vi "Check Trigger.vi"(3 "error in (no error)":errorcluster, 4 "Average Integration\nThreshold (V ms)":dbl(slide)=100.0 scale=0.0..100.0, 5 "Force Trigger":bool, 6 "Signals":waveform(dbl)[](array[waveform])) -> (0 "error out":errorcluster, 1 "Average Raw Signal\n Integration Value":dbl, 2 "Triggered":bool)   [LabVIEW 2013]
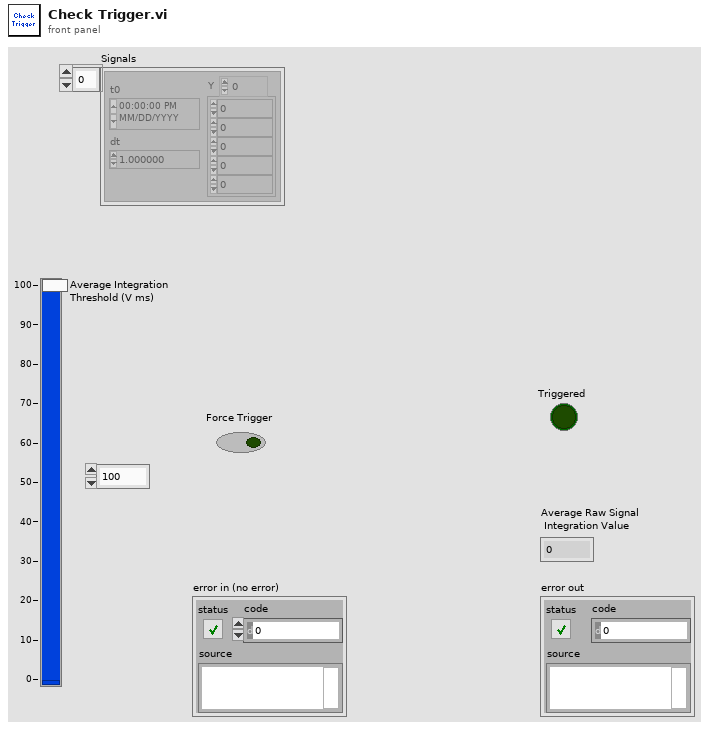
[diagram p1: front panel]
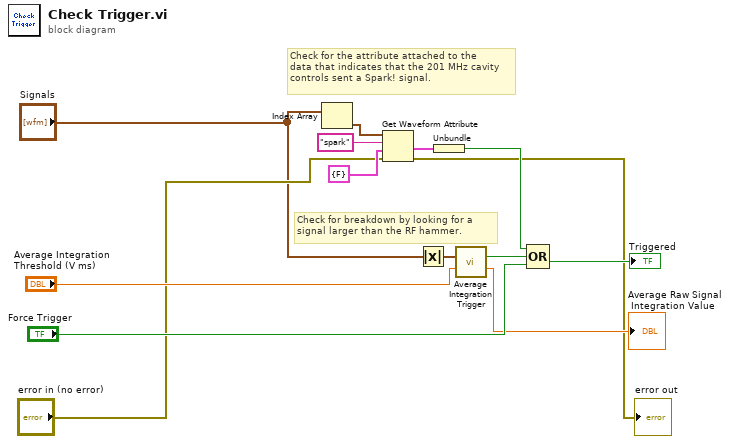
[diagram p0: block diagram]
diagram:
  # "Check for the attribute attached to the\ndata that indicates that the 201 MHz cavity\ncontrols sent a Spark! signal."
  # "Check for breakdown by looking for a\nsignal larger than the RF hammer."
  n1 = Index Array(array="Signals") -> (element=w2:waveform(dbl))  [unwired: 1 in]
  n2 = Get Waveform Attribute(4:"error in (no error)", 5:cluster{bool} {FALSE}, 6:"spark" ("name"), 7:w2) -> (0:→"error out":errorcluster, 1:w7:cluster{bool})  [unwired: 2 out]
  n3 = Absolute Value(x="Signals") -> (abs(x)=w11:waveform(dbl)[])
  n4 = Unbundle(w7) -> (w6:bool)
  n5 = call "Average Integration Trigger.vi"("Waveforms"=w11, "Threshold (V ms)"="Average Integration\nThreshold (V ms)") -> ("Satisfied?"=w10:bool, "Average Integration Value"=→"Average Raw Signal\n Integration Value":dbl)  [unwired: 12 in]
  n6 = Compound Arithmetic op=OR(w6, w10, "Force Trigger") -> (→"Triggered":bool)
